vi "autofocus calibrate.vi"(8 "Error In":errorcluster, 11 "Handle":i32) -> (0 "Error Out":errorcluster, 2 "Intensity OK":bool=TRUE, 3 "Cal. curve":cluster{ext[], dbl[]})   [LabVIEW 2014]
uses:
  Shutter Control/Shutter SubVis/user event shutter global.ctl
  Stage Control/Stage SubVis/move stage.ctl
  autofocus-globals.vi
  tirf-lock-globals.vi
panel:
  out "Calibration curve":cluster{ext[], dbl[]}(graph)
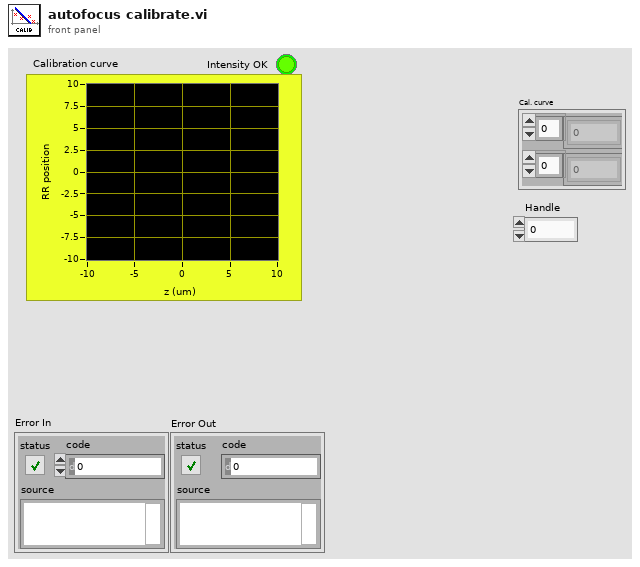
[diagram p1: front panel]
types:
  T1 = enum32{"No Selection", "GFP", "Cy3 Long \nPass", "Cy3", "Cy5", "Off", "IR"}
  T2 = typedef "user event shutter global.ctl" = cluster{"Camera Shutter":bool, "Wheel Speed":u8, "Laser Shutter":enum32{"No Selection", "GFP", "Cy3 Long \nPass", "Cy3", "Cy5", "Off", "IR"}}
  T3 = typedef "move stage.ctl" = cluster{"dx (um) (0 -> ignore)":ext, "dy (um) (0 -> ignore)":ext, "dz (um) (0 -> ignore)":ext, "Re-center x,y":bool, "Re-center z":bool, "x (um) (-1 -> ignore)":dbl, "y (um) (-1 -> ignore)":dbl, "z (um) (-1 -> ignore)":dbl}
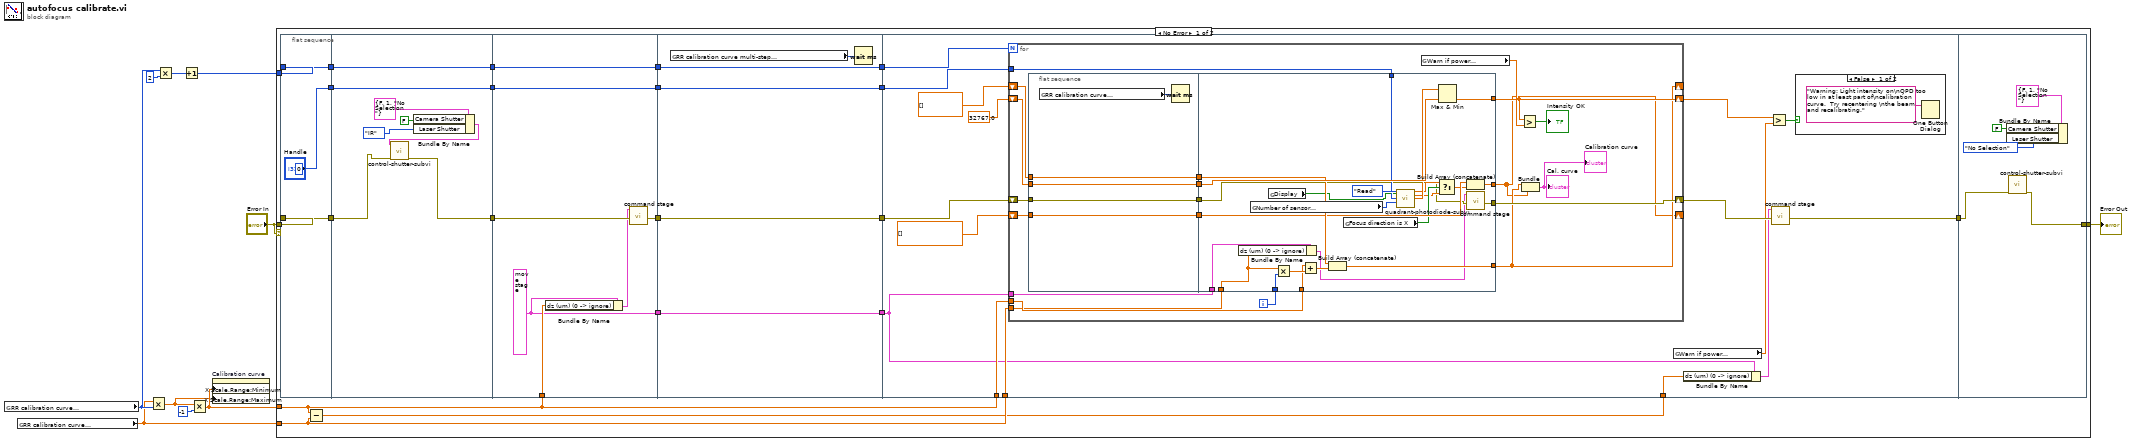
[diagram p0: block diagram]
diagram:
  n1 = global read "autofocus-globals.vi" "RR calibration curve\nhalf-width  (steps)"() -> (w6:u16)
  n2 = global read "autofocus-globals.vi" "RR calibration curve\nstep size (um)"() -> (w3:ext)
  n3 = Multiply(x=w3, y=w6) -> (x*y=w1:ext)
  n4 = Multiply(x=w6, y=2) -> (x*y=w5:i32)
  n5 = Increment(x=w5) -> (x+1=w4:i32)
  n6 = Multiply(x=w1, y=-1) -> (x*y=w2:ext)
  n7 = property on="Calibration curve" class="XYGraph (strict)"("X Scale.Range:Minimum"=w2, "X Scale.Range:Maximum"=w1) -> ()  [unwired: 2 in, 2 out]
  n8 = case shown="No Error" "Error In" {
    tunnel: "Error In" -> [w29 w126]
    tunnel: [w11 w126] -> w9
    tunnel: w2 -> [w19 _]
    tunnel: w4 -> [w31 _]
    tunnel: w3 -> [w18 _]
    frame No Error {
      n9 = flat-sequence {
        tunnel: w31 -> [w33]
        tunnel: [w34] -> w30
        tunnel: w29 -> [w34]
        tunnel: [w33] -> w23
        tunnel: ["Handle"] -> w12
        tunnel: w30 -> [w40]
        tunnel: [w39] -> w28
        tunnel: [w42] -> w24
        tunnel: w23 -> [w42]
        tunnel: [w41] -> w13
        tunnel: w12 -> [w41]
        tunnel: w28 -> [w49]
        tunnel: w19 -> [w47]
        tunnel: [w48] -> w27
        tunnel: [w45] -> w26
        tunnel: [w44] -> w25
        tunnel: w24 -> [w44]
        tunnel: [w43] -> w14
        tunnel: w13 -> [w43]
        tunnel: w27 -> [w54]
        tunnel: w26 -> [w53]
        tunnel: w25 -> [w51]
        tunnel: [w54] -> w22
        tunnel: [w53] -> w21
        tunnel: [w51] -> w20
        tunnel: [w50] -> w15
        tunnel: w14 -> [w50]
        tunnel: w22 -> [w69]
        tunnel: w21 -> [w60]
        tunnel: w20 -> [w70]
        tunnel: w19 -> [w65]
        tunnel: w18 -> [w64]
        tunnel: w17 -> [w62]
        tunnel: [w59] -> w16
        tunnel: w15 -> [w55]
        tunnel: w16 -> [w125]
        tunnel: [w124] -> w11
        frame #0 {
          (unwired) 0
        }
        frame #1 {
          n10 = Bundle By Name(cluster=T2 {"Camera Shutter"=FALSE, "Wheel Speed"=1, "Laser Shutter"=enum."No Selection"} ("Shutter Control"), "Camera Shutter"=FALSE, "Laser Shutter"=T1."IR") -> (w35:T2)
          n11 = call "control-shutter-subvi.vi"("Error In"=w40, "Shutter Control"=w35) -> ("Error Out"=w39:errorcluster)  [unwired: 9 in]
        }
        frame #2 {
          w45 = T3 {"dx (um) (0 -> ignore)"=0.0, "dy (um) (0 -> ignore)"=0.0, "dz (um) (0 -> ignore)"=0.0, "Re-center x,y"=FALSE, "Re-center z"=FALSE, "x (um) (-1 -> ignore)"=-1.0, "y (um) (-1 -> ignore)"=-1.0, "z (um) (-1 -> ignore)"=-1.0} ("Command Stage")
          n12 = Bundle By Name(cluster=w45, "dz (um) (0 -> ignore)"=w47) -> (w46:T3)
          n13 = call "command stage.vi"("Error In"=w49, "Command Stage"=w46) -> ("Error Out"=w48:errorcluster)  [unwired: 9 in]
        }
        frame #3 {
          n14 = global read "autofocus-globals.vi" "RR calibration curve multi-step\nadd'l settle time (ms)"() -> (w52:u16)
          n15 = Wait (ms)(milliseconds to wait=w52) -> ()  [unwired: 1 out]
        }
        frame #4 {
          n16 = for {
            N: w70 -> [_]
            shift-right: [w83] -> w63
            shift-left: w69 -> [w91]
            shift-right: [w76] -> w58
            shift-left: 32767.0 -> [w87]
            shift-right: [w73] -> _
            shift-left: dbl[] [] ("z (um)") -> [w88]
            shift-right: [w72] -> _
            shift-left: dbl[] [] ("QPD position") -> [w89]
            tunnel: w65 -> [w82]
            tunnel: w64 -> [w80]
            tunnel: w60 -> [w79]
            tunnel: w55 -> [w74]
            i -> [w81]
            n17 = flat-sequence {
              tunnel: w91 -> [w95]
              tunnel: [w95] -> w90
              tunnel: w89 -> [w94]
              tunnel: w88 -> [w93]
              tunnel: w87 -> [w92]
              tunnel: [w94] -> w86
              tunnel: [w93] -> w85
              tunnel: [w92] -> w84
              tunnel: w90 -> [w99]
              tunnel: w86 -> [w113]
              tunnel: w85 -> [w114]
              tunnel: w84 -> [w116]
              tunnel: [w118] -> w83
              tunnel: w82 -> [w117]
              tunnel: [w115] -> w76
              tunnel: [w111] -> w72
              tunnel: w81 -> [w110]
              tunnel: w80 -> [w109]
              tunnel: w79 -> [w108]
              tunnel: [w106] -> w73
              tunnel: w74 -> [w101]
              frame #0 {
                n18 = global read "autofocus-globals.vi" "RR calibration curve\nsettle time (ms)"() -> (w96:u16)
                n19 = Wait (ms)(milliseconds to wait=w96) -> ()  [unwired: 1 out]
              }
              frame #1 {
                n20 = Bundle By Name(cluster=w108, "dz (um) (0 -> ignore)"=w109) -> (w97:T3)
                n21 = global read "autofocus-globals.vi" "Number of sensor\nreadings to average"() -> (w100:i32)
                n22 = global read "tirf-lock-globals.vi" "Display"() -> (w98:bool)
                n23 = Multiply(x=w109, y=w110) -> (x*y=w120:ext)
                n24 = Add(x=w117, y=w120) -> (x+y=w119:ext)
                n25 = Build Array (concatenate)(w114, w119) -> (w106:ext[])
                n26 = global read "autofocus-globals.vi" "Focus direction is X"() -> (w107:bool)
                n27 = call "quadrant-photodiode-subvi.vi"("Mode"=enum16{"Start", "Read", "End"}."Read", "Display"=w98, "Handle"=w101, "Averages"=w100) -> ("coerced(x)"=w102:dbl, "coerced(y)"=w103:dbl, "Power (mw)"=w104:dbl)  [unwired: 9 in]
                n28 = Select(t=w102, s=w107, f=w103) -> (s? t:f=w112:dbl)
                n29 = Max & Min(x=w104, y=w116) -> (min(x,y)=w115:dbl)  [unwired: 1 out]
                n30 = Build Array (concatenate)(w113, w112) -> (w111:dbl[])
                n31 = call "command stage.vi"("Error In"=w99, "Command Stage"=w97) -> ("Error Out"=w118:errorcluster)  [unwired: 9 in]
              }
            }
            n32 = global read "autofocus-globals.vi" "Warn if power \nless than"() -> (w77:dbl)
            n33 = Greater?(x=w76, y=w77) -> (0:→"Intensity OK":bool)
            n34 = Bundle(w73, w72) -> (→"Cal. curve" →"Calibration curve":cluster{ext[], dbl[]})  [unwired: 1 in]
          }
          n35 = global read "autofocus-globals.vi" "Warn if power \nless than"() -> (w57:dbl)
          n36 = Bundle By Name(cluster=w60, "dz (um) (0 -> ignore)"=w62) -> (w61:T3)
          n37 = Greater?(x=w58, y=w57) -> (0:w56:bool)
          n38 = call "command stage.vi"("Error In"=w63, "Command Stage"=w61) -> ("Error Out"=w59:errorcluster)  [unwired: 9 in]
          n39 = case shown="False" w56 {
            frame False {
              n40 = One Button Dialog(message="Warning: Light intensity on\nQPD too low in at least part of\ncalibration curve.  Try recentering \nthe beam and recalibrating.") -> ()  [unwired: 2 out]
            }
            frame True {
            }
          }
        }
        frame #5 {
          n41 = Bundle By Name(cluster=T2 {"Camera Shutter"=FALSE, "Wheel Speed"=1, "Laser Shutter"=enum."No Selection"} ("Shutter Control"), "Camera Shutter"=FALSE, "Laser Shutter"=T1."No Selection") -> ()  [unwired: 1 out]
          n42 = call "control-shutter-subvi.vi"("Error In"=w125) -> ("Error Out"=w124:errorcluster)  [unwired: 10 in]
        }
      }
      n43 = Subtract(x=w19, y=w18) -> (x-y=w17:ext)
    }
    frame Error {
    }
  }
  "Error Out" <- w9
